vi "Assign booleans from string to axes.vi"(0 "System no.":i32=1 min=1 max=4 step=1, 2 "Queried axes":string[](array[string]), 3 "All axes queried?":bool, 4 "Input String":string, 5 "error in":errorcluster) -> (14 "Booleans":bool[](array[boolean]), 19 "error out":errorcluster)   [LabVIEW 2020]
doc: "This VI assigns numerical values from input string to boolean values for queried axes. If All axes is TRUE, connected axes are read from Global2.vi and displayed on the front panel for assignment. \nExample: An input string like \"A=0SpaceLinefeedB=1Linefeed\" or \"0SpaceLinefeed1Linefeed\" will be converted to an output array consisting of two values \"FALSE; TRUE\"."
panel:
  # "This vi assigns values from input string to boolean values for queried axes. If \"All axes\" is true, connected axes are read from Global2.vi"
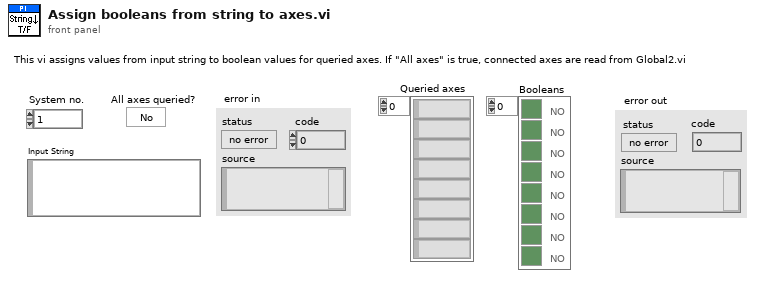
[diagram p1: front panel]
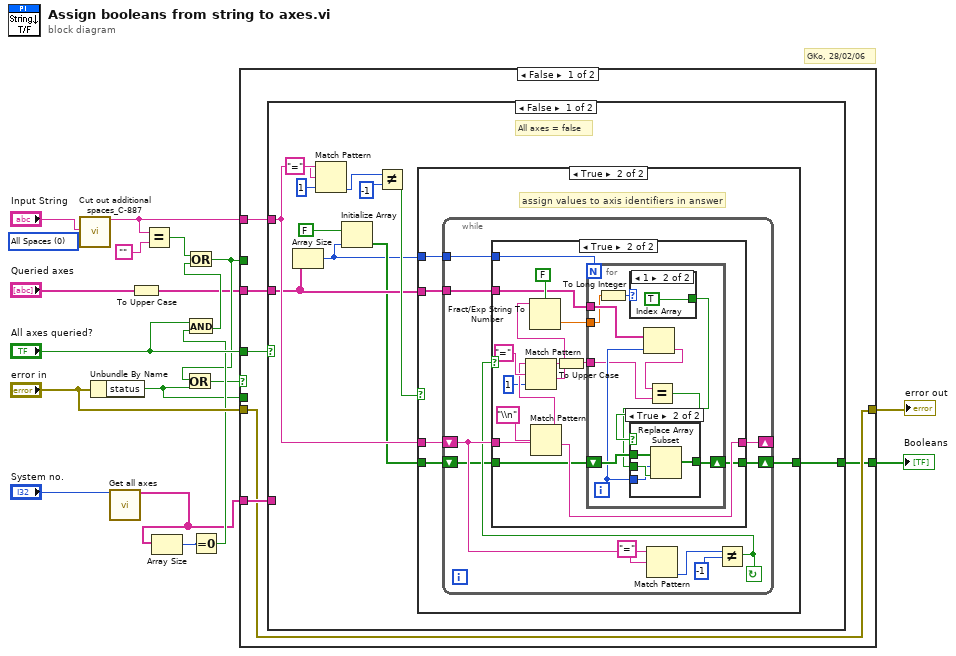
[diagram p0: block diagram]
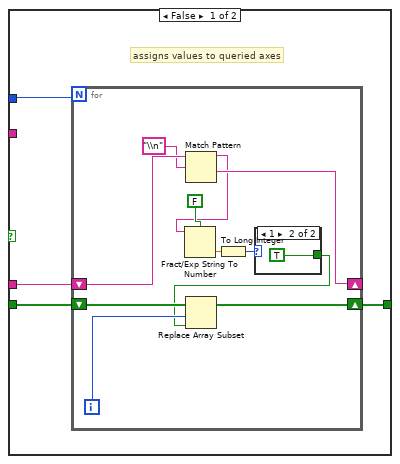
[diagram p2: hidden frame]
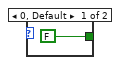
[diagram p3: hidden frame]
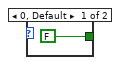
[diagram p5: hidden frame]
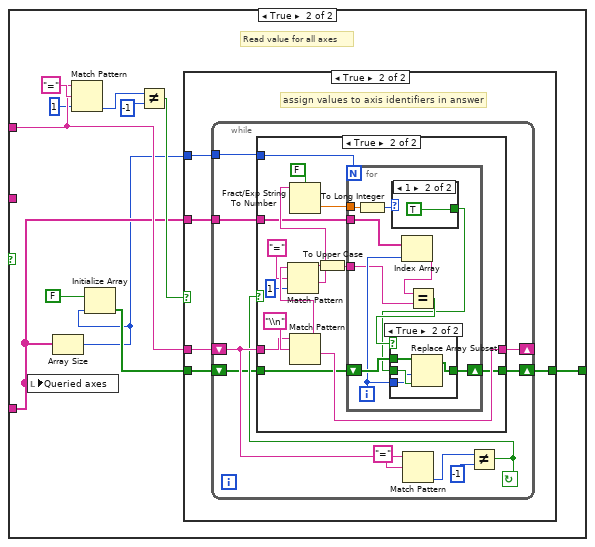
[diagram p7: hidden frame]
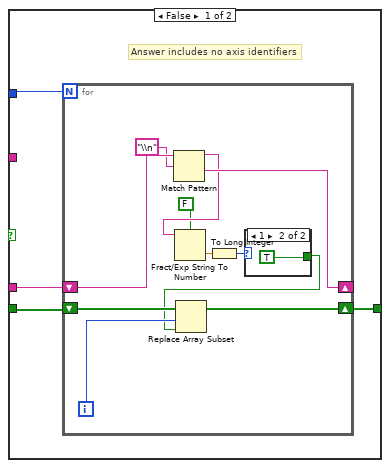
[diagram p8: hidden frame]
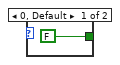
[diagram p9: hidden frame]
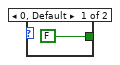
[diagram p11: hidden frame]
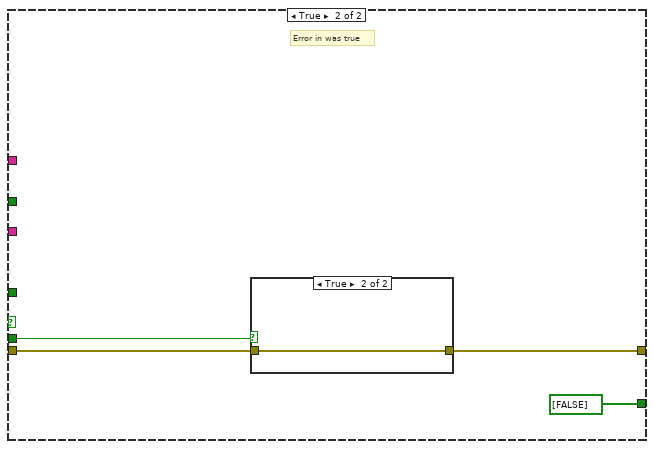
[diagram p13: hidden frame]
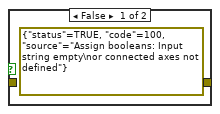
[diagram p14: hidden frame]
diagram:
  w1 = u16 0 items=["All Spaces", "Only if 1st char.", "Only if last char.", "Only if near \"=\""] ("Mode")
  # "GKo, 28/02/06"
  n1 = call "Cut out additional spaces_C-887.vi"("String"="Input String", "Mode"=w1) -> ("String out"=w3:string)  [unwired: 17 out]
  n2 = Unbundle By Name("error in") -> ("status"=w6:bool)
  n3 = call "Get all axes.vi"("System no."="System no.") -> ("Conn. Axes"=w4:string[])  [unwired: 18 out]
  n4 = To Upper Case(1:"Queried axes") -> (0:w7:string[])
  n5 = Equal?(x=w3, y="") -> (x = y?=w15:bool)
  n6 = Array Size(array=w4) -> (size(s)=w13:i32)
  n7 = Equal To 0?(x=w13) -> (x = 0?=w12:bool)
  n8 = And(x="All axes queried?", y=w12) -> (x .and. y?=w11:bool)
  n9 = Or(x=w15, y=w11) -> (x .or. y?=w9:bool)
  n10 = Or(x=w9, y=w6) -> (x .or. y?=w10:bool)
  n11 = case shown="False" w10 {
    tunnel: "All axes queried?" -> [w25 _]
    tunnel: w3 -> [w24 _]
    tunnel: [w20 bool[] [FALSE] ("Axis on target?")] -> w8
    tunnel: w7 -> [w23 _]
    tunnel: w4 -> [w22 _]
    tunnel: [w21 w182] -> w17
    tunnel: "error in" -> [w21 w183]
    tunnel: w9 -> [_ _]
    tunnel: w6 -> [_ w180]
    frame False {
      n12 = case shown="False" w25 {
        tunnel: w24 -> [w35 w109]
        tunnel: [w36 w113] -> w20
        tunnel: w23 -> [w30 _]
        tunnel: w22 -> [_ w106]
        frame False {
          # "All axes = false"
          n13 = Array Size(array=w30) -> (size(s)=w28:i32)
          n14 = Match Pattern(string=w35, regular expression="=", offset (0)=1) -> (offset past match=w32:i32)  [unwired: 3 out]
          n15 = Initialize Array(FALSE, w28) -> (w29:bool[])
          n16 = Not Equal?(x=w32, y=-1) -> (x != y?=w31:bool)
          n17 = case shown="True" w31 {
            tunnel: [w40 w57] -> w36
            tunnel: w35 -> [w39 w58]
            tunnel: w30 -> [_ w56]
            tunnel: w29 -> [w38 w54]
            tunnel: w28 -> [w37 w55]
            frame False {
              # "assigns values to queried axes"
              n18 = for {
                N: w37 -> [_]
                shift-right: [w44] -> w40
                shift-left: w38 -> [w45]
                shift-right: [w50] -> _
                shift-left: w39 -> [w51]
                i -> [w46]
                n19 = Match Pattern(string=w51, regular expression="\\n") -> (before substring=w47:string, after substring=w50:string)  [unwired: 3 out]
                n20 = Fract/Exp String To Number(use system decimal point (T)=FALSE, string=w47) -> (number=w43:dbl)  [unwired: 3 out]
                n21 = To Long Integer(number=w43) -> (32bit integer=w41:i32)
                n22 = case shown="1" w41 {
                  tunnel: [FALSE TRUE] -> w42
                  frame 0, Default {
                  }
                  frame 1 {
                  }
                }
                n23 = Replace Array Subset(array=w45, new element=w42, index=w46) -> (w44:bool[])
              }
            }
            frame True {
              # "assign values to axis identifiers in answer"
              n24 = while {
                tunnel: w55 -> [w59]
                tunnel: w56 -> [w60]
                shift-left: w54 -> [w62]
                shift-right: [w61] -> w57
                shift-left: w58 -> [w65]
                shift-right: [w64] -> _
                stop <- w63 continue-if-true
                n25 = Match Pattern(string=w65, regular expression="=") -> (offset past match=w66:i32)  [unwired: 4 out]
                n26 = Not Equal?(x=w66, y=-1) -> (x != y?=w63:bool)
                n27 = case shown="True" w63 {
                  tunnel: w65 -> [w70 w84]
                  tunnel: [w70 w83] -> w64
                  tunnel: [w69 w81] -> w61
                  tunnel: w62 -> [w69 w82]
                  tunnel: w60 -> [_ w75]
                  tunnel: w59 -> [_ w73]
                  frame False {
                  }
                  frame True {
                    n28 = Match Pattern(string=w84, regular expression="\\n") -> (before substring=w77:string, after substring=w83:string)  [unwired: 3 out]
                    n29 = Match Pattern(string=w77, regular expression="=", offset (0)=1) -> (before substring=w74:string, after substring=w79:string)  [unwired: 2 out]
                    n30 = Fract/Exp String To Number(use system decimal point (T)=FALSE, string=w79) -> (number=w76:dbl)  [unwired: 3 out]
                    n31 = To Upper Case(1:w74) -> (0:w71:string)
                    n32 = for {
                      N: w73 -> [_]
                      tunnel: w76 -> [w88]
                      shift-right: [w94] -> w81
                      shift-left: w82 -> [w95]
                      tunnel: w75 -> [w92]
                      tunnel: w71 -> [w90]
                      i -> [w93]
                      n33 = To Long Integer(number=w88) -> (32bit integer=w86:i32)
                      n34 = case shown="1" w86 {
                        tunnel: [FALSE TRUE] -> w87
                        frame 0, Default {
                        }
                        frame 1 {
                        }
                      }
                      n35 = Index Array(array=w92, index=w93) -> (element=w91:string)
                      n36 = Equal?(x=w91, y=w90) -> (x = y?=w89:bool)
                      n37 = case shown="True" w89 {
                        tunnel: w87 -> [_ w102]
                        tunnel: w93 -> [_ w99]
                        tunnel: w95 -> [w98 w101]
                        tunnel: [w98 w100] -> w94
                        frame False {
                        }
                        frame True {
                          n38 = Replace Array Subset(array=w101, new element=w102, index=w99) -> (w100:bool[])
                        }
                      }
                    }
                  }
                }
              }
            }
          }
        }
        frame True {
          # "Read value for all axes"
          n39 = local write "Queried axes"(w106) -> ()
          n40 = Array Size(array=w106) -> (size(s)=w105:i32)
          n41 = Match Pattern(string=w109, regular expression="=", offset (0)=1) -> (offset past match=w110:i32)  [unwired: 3 out]
          n42 = Initialize Array(FALSE, w105) -> (w107:bool[])
          n43 = Not Equal?(x=w110, y=-1) -> (x != y?=w108:bool)
          n44 = case shown="True" w108 {
            tunnel: [w117 w135] -> w113
            tunnel: w109 -> [w116 w134]
            tunnel: w106 -> [_ w133]
            tunnel: w107 -> [w115 w132]
            tunnel: w105 -> [w114 w131]
            frame False {
              # "Answer includes no axis identifiers"
              n45 = for {
                N: w114 -> [_]
                shift-right: [w124] -> w117
                shift-left: w115 -> [w126]
                shift-right: [w127] -> _
                shift-left: w116 -> [w128]
                i -> [w125]
                n46 = Match Pattern(string=w128, regular expression="\\n") -> (before substring=w122:string, after substring=w127:string)  [unwired: 3 out]
                n47 = Fract/Exp String To Number(use system decimal point (T)=FALSE, string=w122) -> (number=w120:dbl)  [unwired: 3 out]
                n48 = To Long Integer(number=w120) -> (32bit integer=w118:i32)
                n49 = case shown="1" w118 {
                  tunnel: [FALSE TRUE] -> w119
                  frame 0, Default {
                  }
                  frame 1 {
                  }
                }
                n50 = Replace Array Subset(array=w126, new element=w119, index=w125) -> (w124:bool[])
              }
            }
            frame True {
              # "assign values to axis identifiers in answer"
              n51 = while {
                tunnel: w131 -> [w136]
                tunnel: w133 -> [w137]
                shift-left: w132 -> [w139]
                shift-right: [w138] -> w135
                shift-left: w134 -> [w142]
                shift-right: [w141] -> _
                stop <- w140 continue-if-true
                n52 = Match Pattern(string=w142, regular expression="=") -> (offset past match=w143:i32)  [unwired: 4 out]
                n53 = Not Equal?(x=w143, y=-1) -> (x != y?=w140:bool)
                n54 = case shown="True" w140 {
                  tunnel: w142 -> [w147 w161]
                  tunnel: [w147 w160] -> w141
                  tunnel: [w146 w158] -> w138
                  tunnel: w139 -> [w146 w159]
                  tunnel: w137 -> [_ w151]
                  tunnel: w136 -> [_ w150]
                  frame False {
                  }
                  frame True {
                    n55 = Match Pattern(string=w161, regular expression="\\n") -> (before substring=w157:string, after substring=w160:string)  [unwired: 3 out]
                    n56 = Match Pattern(string=w157, regular expression="=", offset (0)=1) -> (before substring=w155:string, after substring=w154:string)  [unwired: 2 out]
                    n57 = Fract/Exp String To Number(use system decimal point (T)=FALSE, string=w154) -> (number=w153:dbl)  [unwired: 3 out]
                    n58 = To Upper Case(1:w155) -> (0:w148:string)
                    n59 = for {
                      N: w150 -> [_]
                      tunnel: w148 -> [w167]
                      tunnel: w153 -> [w165]
                      shift-right: [w171] -> w158
                      shift-left: w159 -> [w172]
                      tunnel: w151 -> [w170]
                      i -> [w169]
                      n60 = To Long Integer(number=w165) -> (32bit integer=w163:i32)
                      n61 = case shown="1" w163 {
                        tunnel: [FALSE TRUE] -> w164
                        frame 0, Default {
                        }
                        frame 1 {
                        }
                      }
                      n62 = Index Array(array=w170, index=w169) -> (element=w168:string)
                      n63 = Equal?(x=w168, y=w167) -> (x = y?=w166:bool)
                      n64 = case shown="True" w166 {
                        tunnel: w164 -> [_ w179]
                        tunnel: w169 -> [_ w176]
                        tunnel: w172 -> [w175 w178]
                        tunnel: [w175 w177] -> w171
                        frame False {
                        }
                        frame True {
                          n65 = Replace Array Subset(array=w178, new element=w179, index=w176) -> (w177:bool[])
                        }
                      }
                    }
                  }
                }
              }
            }
          }
        }
      }
    }
    frame True {
      # "Error in was true"
      n66 = case shown="True" w180 {
        tunnel: w183 -> [_ w185]
        tunnel: [errorcluster {"status"=TRUE, "code"=100, "source"="Assign booleans: Input string empty\nor connected axes not defined"} ("error out") w185] -> w182
        frame False {
        }
        frame True {
        }
      }
    }
  }
  "Booleans" <- w8
  "error out" <- w17
